vi "AVI filepath manager.vi"(8 "error in (no error)":errorcluster) -> (0 "error":errorcluster, 1 "AVI File Path":path, 3 "File path OK":bool)   [LabVIEW 2017]
uses:
  Globals/gl_Time series viewer globals.vi
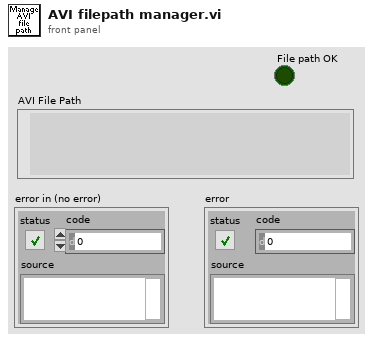
[diagram p1: front panel]
types:
  T1 = typedef "Time series viewer refs.ctl" = cluster{"This VI":refnum<vi>, "Image control":refnum<vi>, "AVI Mode ind":refnum<vi>, "Play":refnum<vi>, "Stop":refnum<vi>, "Back":refnum<vi>, "Scrollbar":refnum<vi>, "Video length info":refnum<vi>, "Expected speed values":refnum<vi>, "Intensity":refnum<vi>, "Path":refnum<vi>, "Selection sliders":refnum<vi>, "Speed Graph ref":refnum<vi>, "Frame rate set (fps)":refnum<vi>, "Channel to load":refnum<vi>, "Number of rows to generate":refnum<vi>, "Colour":refnum<vi>}
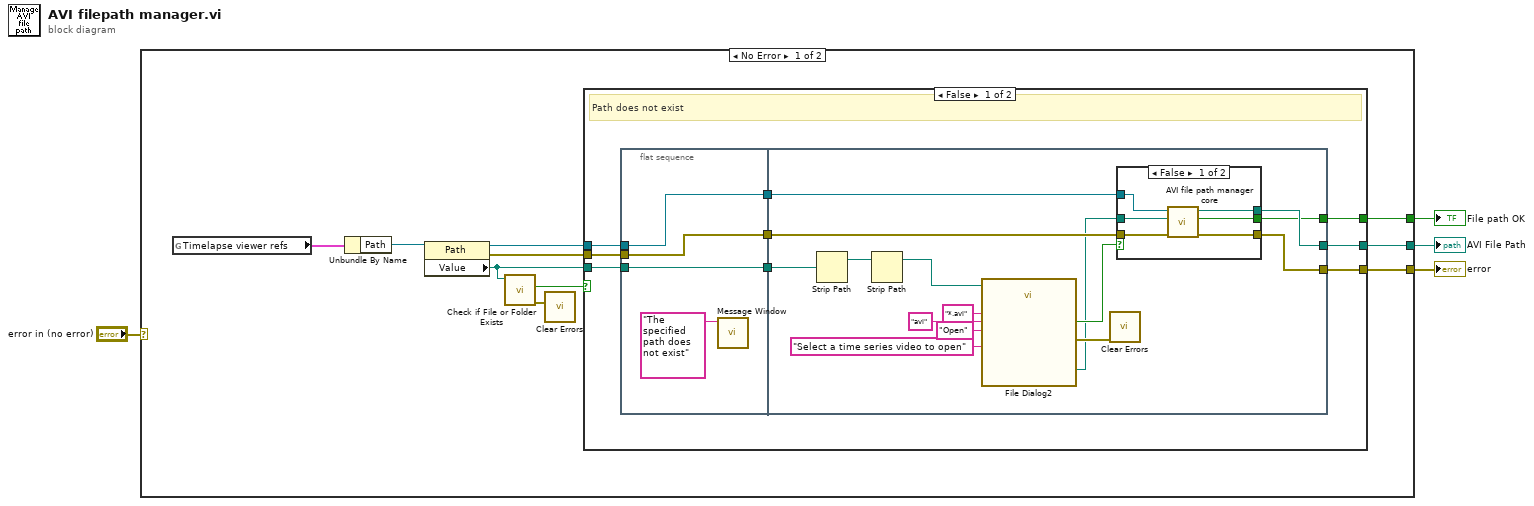
[diagram p0: block diagram]
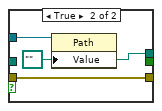
[diagram p2: hidden frame]
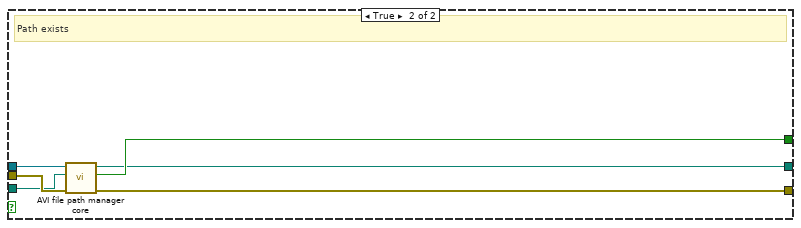
[diagram p3: hidden frame]
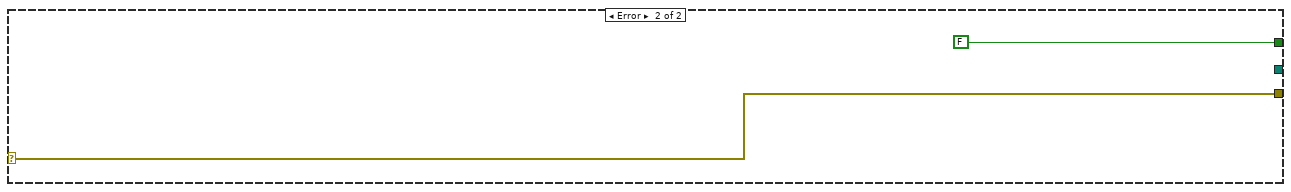
[diagram p4: hidden frame]
diagram:
  n1 = case shown="No Error" "error in (no error)" {
    selector: "error in (no error)" -> [_ w58]
    tunnel: [w12 FALSE ("File path OK 2")] -> w4
    tunnel: [w10 _] -> w3
    tunnel: [w8 w58] -> w1
    frame No Error {
      n2 = global read "gl_Time series viewer globals.vi" "Timelapse viewer refs"() -> (w13:T1)
      n3 = Unbundle By Name(w13) -> ("Path"=w14:refnum<vi>)
      n4 = property class="Path"(reference=w14) -> (reference out=w11:refnum<vi>, error out=w9:errorcluster, "Value"=w7:path)  [unwired: 1 in]
      n5 = call <vilib>:"Check if File or Folder Exists.vi"("path"=w7) -> ("error out"=w5:errorcluster, "file or folder exists?"=w6:bool)  [unwired: 8 in, 1 out]
      n6 = call <vilib>:"Clear Errors.vi"("error in (no error)"=w5) -> ()  [unwired: 5 in, 2 out]
      n7 = case shown="False" w6 {
        tunnel: [w15 w57] -> w12
        tunnel: w11 -> [w20 w56]
        tunnel: [w23 w55] -> w10
        tunnel: w9 -> [w17 w54]
        tunnel: [w16 w53] -> w8
        tunnel: w7 -> [w21 w52]
        frame False {
          # "Path does not exist"
          n8 = flat-sequence {
            tunnel: [w26] -> w22
            tunnel: w21 -> [w26]
            tunnel: w20 -> [w25]
            tunnel: [w25] -> w19
            tunnel: [w24] -> w18
            tunnel: w17 -> [w24]
            tunnel: [w29] -> w23
            tunnel: w22 -> [w37]
            tunnel: w19 -> [w33]
            tunnel: w18 -> [w32]
            tunnel: [w31] -> w16
            tunnel: [w28] -> w15
            frame #0 {
              n9 = call "Message Window.vi"("Message string"="The specified path does not exist") -> ()  [unwired: 10 in, 1 out]
            }
            frame #1 {
              n10 = Strip Path(path=w37) -> (stripped path=w36:path)  [unwired: 1 out]
              n11 = Strip Path(path=w36) -> (stripped path=w35:path)  [unwired: 1 out]
              n12 = call "File Dialog2"("start path"=w35, "prompt"="Select a time series video to open", "button label"="Open", "pattern (all files)"="*.avi", "pattern label"="avi") -> ("selected path"=w30:path, "cancelled"=w34:bool, "error out"=w39:errorcluster)  [unwired: 7 in, 1 out]
              n13 = call <vilib>:"Clear Errors.vi"("error in (no error)"=w39) -> ()  [unwired: 5 in, 2 out]
              n14 = case shown="False" w34 {
                tunnel: w30 -> [w45 _]
                tunnel: w33 -> [w48 w50]
                tunnel: w32 -> [w47 w51]
                tunnel: [w46 w51] -> w31
                tunnel: [w44 w49] -> w29
                tunnel: [w43 _] -> w28
                frame False {
                  n15 = call "AVI file path manager core.vi"("error in (no error)"=w47, "Value in"=w45, "Path in"=w48) -> ("error out"=w46:errorcluster, "File path OK"=w43:bool, "File path"=w44:path)  [unwired: 6 in]
                }
                frame True {
                  w49 = path "" ("Value")
                  n16 = property class="Path"(reference=w50, "Value"=w49) -> ()  [unwired: 1 in, 2 out]
                }
              }
            }
          }
        }
        frame True {
          # "Path exists"
          n17 = call "AVI file path manager core.vi"("error in (no error)"=w54, "Value in"=w52, "Path in"=w56) -> ("error out"=w53:errorcluster, "File path OK"=w57:bool, "File path"=w55:path)  [unwired: 6 in]
        }
      }
    }
    frame Error {
    }
  }
  "File path OK" <- w4
  "AVI File Path" <- w3
  "error" <- w1
